vi "sv_Generate Discrete Steps.vi"(8 "error in (no error)":errorcluster, 9 "spacing":enum16{"linear", "logarithmic"}(ring), 10 "steps":cluster{"start":dbl, "stop":dbl, "number":i32}={"start"=20.0, "stop"=20000.0, "number"=100} {"stop" min=0.0 format="%.2f"; "start" min=0.0 format="%.2f"}) -> (0 "error out":errorcluster, 1 "frequency list":dbl[](array[numeric]) format="%.2f")   [LabVIEW 2017]
uses:
  <vilib>/Analysis/1siggen.llb/Ramp Pattern by Samples.vi
  <vilib>/Analysis/NI_AALBase.lvlib
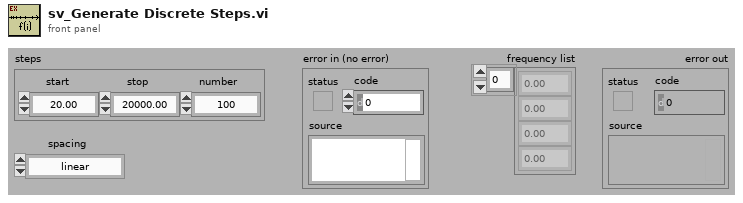
[diagram p1: front panel]
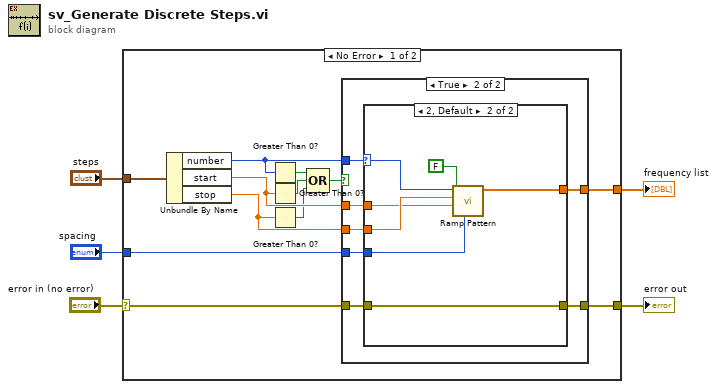
[diagram p0: block diagram]
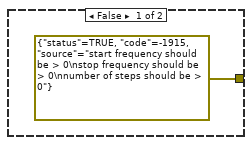
[diagram p2: hidden frame]
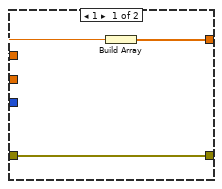
[diagram p3: hidden frame]
diagram:
  n1 = case shown="No Error" "error in (no error)" {
    selector: "error in (no error)" -> [w16 w36]
    tunnel: "steps" -> [w17 _]
    tunnel: "spacing" -> [w15 _]
    tunnel: [w13 _] -> w4
    tunnel: [w12 w36] -> w2
    frame No Error {
      n2 = Unbundle By Name(w17) -> ("number"=w10:i32, "start"=w14:dbl, "stop"=w11:dbl)
      n3 = Greater Than 0?(x=w10) -> (x > 0?=w9:bool)
      n4 = Greater Than 0?(x=w14) -> (x > 0?=w8:bool)
      n5 = Greater Than 0?(x=w11) -> (x > 0?=w7:bool)
      n6 = Compound Arithmetic op=OR(w9, w8, w7) -> (w6:bool)
      n7 = case shown="True" w6 {
        tunnel: w16 -> [_ w22]
        tunnel: w15 -> [_ w25]
        tunnel: w14 -> [_ w24]
        tunnel: [_ w23] -> w13
        tunnel: [errorcluster {"status"=TRUE, "code"=-1915, "source"="start frequency should be > 0\nstop frequency should be > 0\nnumber of steps should be > 0"} ("error IO") w21] -> w12
        tunnel: w10 -> [_ w20]
        tunnel: w11 -> [_ w19]
        frame False {
        }
        frame True {
          n8 = case shown="2, Default" w20 {
            selector: w20 -> [_ w33]
            tunnel: w25 -> [_ w30]
            tunnel: w24 -> [w28 w34]
            tunnel: w19 -> [_ w35]
            tunnel: [w27 w32] -> w23
            tunnel: w22 -> [w26 w31]
            tunnel: [w26 w31] -> w21
            frame 1 {
              n9 = Build Array(w28) -> (w27:dbl[])
            }
            frame 2, Default {
              n10 = call-poly <vilib>:"Ramp Pattern.vi"("type"=w30, "exclude end?"=FALSE, "start"=w34, "end"=w35, "samples"=w33) -> ("Ramp Pattern"=w32:dbl[])  [unwired: 5 in, 1 out]
            }
          }
        }
      }
    }
    frame Error {
    }
  }
  "frequency list" <- w4
  "error out" <- w2
